vi "I2S RECDAT In(David Documentation).vi"(0 "I2S.RECLRC IN":bool, 5 "I2S.RECDAT IN":bool, 7 "Data Index":u16, 9 "Bit Count":u16, 11 "Word Length":u16) -> (4 "Data Channel":bool, 15 "Audio Signals":T1)   [LabVIEW 2015]
uses:
  Audio Signals.ctl
panel:
  # "Overview: Read each audio bit from RECDAT pin."
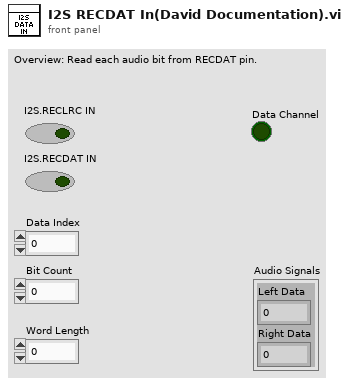
[diagram p1: front panel]
types:
  T1 = typedef "Audio Signals.ctl" = cluster{"Left Data":u32, "Right Data":u32}
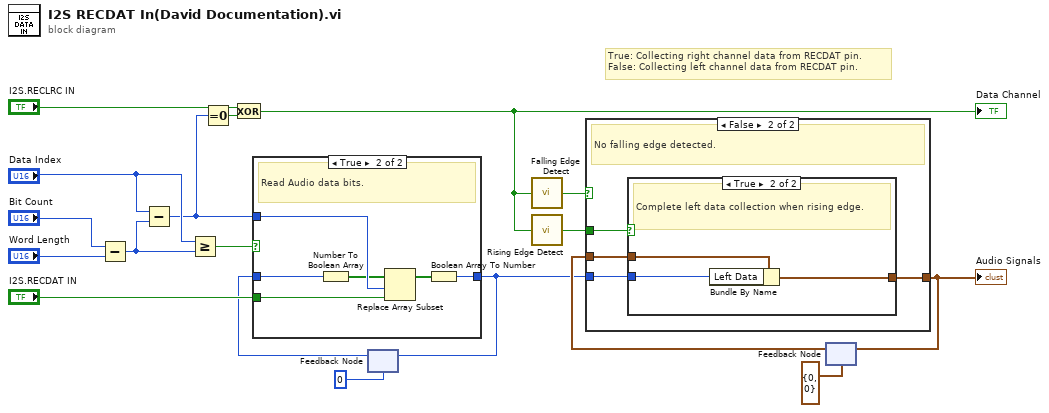
[diagram p0: block diagram]
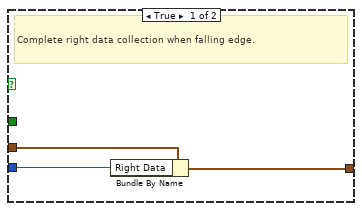
[diagram p2: hidden frame]
diagram:
  # "True: Collecting right channel data from RECDAT pin.\nFalse: Collecting left channel data from RECDAT pin."
  n1 = Subtract(x="Bit Count", y="Word Length") -> (x-y=w10:u16)
  n2 = Subtract(x="Data Index", y=w10) -> (x-y=w13:u16)
  n3 = Greater Or Equal?(x="Data Index", y=w10) -> (x >= y?=w16:bool)
  n4 = Equal To 0?(x=w13) -> (x = 0?=w15:bool)
  n5 = Exclusive Or(1:w15, 2:"I2S.RECLRC IN") -> (0:w3:bool)
  "Data Channel" <- w3
  n6 = feedback #1(u32 0 ("Data In")) -> (w1:u32)
  n7 = case shown="True" w16 {
    tunnel: w13 -> [_ w25]
    tunnel: "I2S.RECDAT IN" -> [_ w24]
    tunnel: [w19 w22] -> w5
    tunnel: w1 -> [w19 w23]
    frame False {
      # "Skip useless bits."
    }
    frame True {
      # "Read Audio data bits."
      n8 = Number To Boolean Array(number=w23) -> (Boolean array=w21:bool[])
      n9 = Replace Array Subset(array=w21, new element=w24, index=w25) -> (w20:bool[])
      n10 = Boolean Array To Number(Boolean array=w20) -> (number=w22:u32)
    }
  }
  n11 = feedback-in #1(w5) -> ()
  n12 = call "Falling Edge Detect.vi"("Signal"=w3) -> ("Trigger?"=w4:bool)
  n13 = call "Rising Edge Detect.vi"("Signal"=w3) -> ("Trigger?"=w2:bool)
  n14 = feedback #2(T1 {"Left Data"=0, "Right Data"=0} ("Audio Signals")) -> (w7:T1)
  n15 = case shown="False" w4 {
    tunnel: w7 -> [w27 w32]
    tunnel: [w26 w31] -> w6
    tunnel: w5 -> [w28 w30]
    tunnel: w2 -> [_ w29]
    frame True {
      # "Complete right data collection when falling edge."
      n16 = Bundle By Name(cluster=w27, "Right Data"=w28) -> (w26:T1)
    }
    frame False {
      # "No falling edge detected."
      n17 = case shown="True" w29 {
        tunnel: w32 -> [w33 w35]
        tunnel: [w33 w36] -> w31
        tunnel: w30 -> [_ w34]
        frame False {
          # "No rising edge detected."
        }
        frame True {
          # "Complete left data collection when rising edge."
          n18 = Bundle By Name(cluster=w35, "Left Data"=w34) -> (w36:T1)
        }
      }
    }
  }
  "Audio Signals" <- w6
  n19 = feedback-in #2(w6) -> ()
